vi "result.vi"() -> ()   [LabVIEW 2013]
uses:
  <vilib>/Utility/file.llb/Read From Spreadsheet File (string).vi
panel:
  out "size(s)":i32
  out "Hours":dbl[](graph)
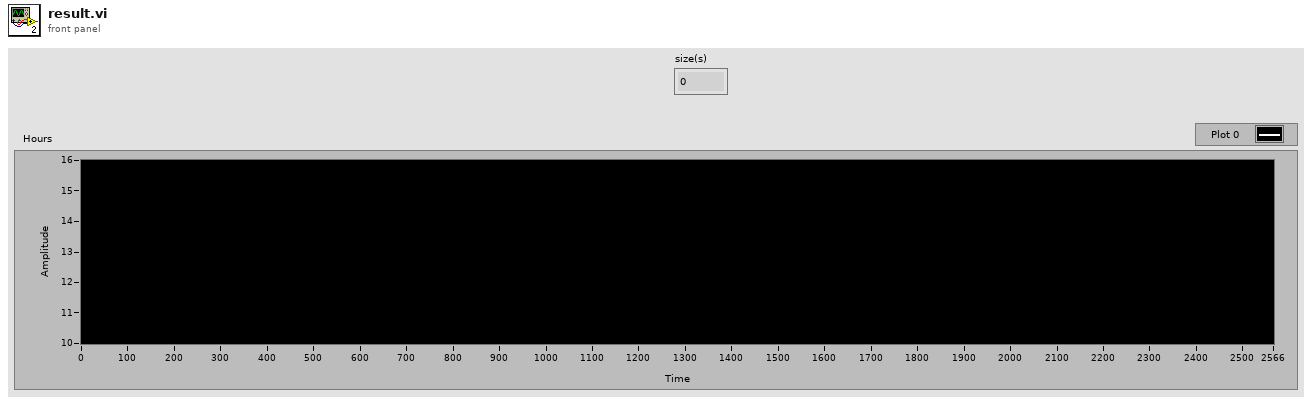
[diagram p1: front panel]
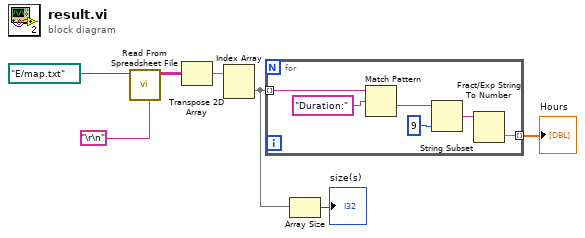
[diagram p0: block diagram]
diagram:
  n1 = call-poly <vilib>:"Read From Spreadsheet File.vi"("delimiter (\\t)"="\r\n", "file path (dialog if empty)"=path "E:/map.txt" ("file (use dialog)")) -> ("all rows"=w5:string[][])  [unwired: 5 in, 4 out]
  n2 = Transpose 2D Array(2D array=w5) -> (transposed array=w4:string[][])
  n3 = Index Array(array=w4) -> (element=w3:string[])  [unwired: 2 in]
  n4 = for {
    tunnel: w3 -> [w13] mode=indexing
    tunnel: [w8] -> w1 mode=indexing
    n5 = Match Pattern(string=w13, regular expression="Duration:") -> (after substring=w11:string)  [unwired: 1 in, 3 out]
    n6 = String Subset(string=w11, length (rest)=9 ("length (rest)")) -> (substring=w9:string)  [unwired: 1 in]
    n7 = Fract/Exp String To Number(string=w9) -> (number=w8:dbl)  [unwired: 3 in, 1 out]
  }
  "Hours" <- w1
  n8 = Array Size(array=w3) -> (size(s)=→"size(s)":i32)
